vi "Reduce Samples.vi"() -> ()   [LabVIEW 2011]
panel:
  in  "stop":bool
  out "Sine":dynamicdata(graph)
  in  "Enable":bool=TRUE
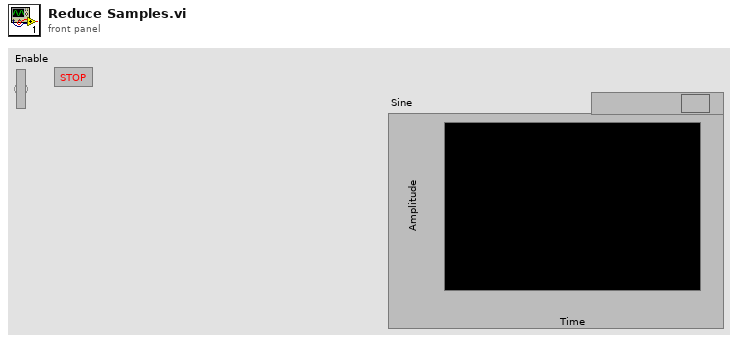
[diagram p1: front panel]
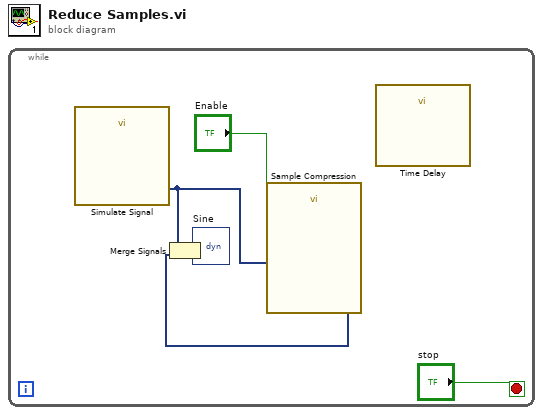
[diagram p0: block diagram]
diagram:
  n1 = while {
    stop <- "stop" stop-if-true
    n2 = call "Simulate Signal"() -> ("Sine"=w5:dynamicdata)  [unwired: 14 in, 1 out]
    n3 = call "Sample Compression"("Enable"="Enable", "Signals"=w5) -> ("Mean"=w2:dynamicdata)  [unwired: 7 in, 2 out]
    n4 = Merge Signals(w5, w2) -> (→"Sine":dynamicdata)
    n5 = call "Time Delay"() -> ()  [unwired: 11 in, 1 out]
  }
